vi "AuMT8852B Single Payload Use Dirty Tx.vi"(5 "Use Dirty transmitter? (F)":bool, 7 "Set/Get (Set)":enum16{"Set", "Get"}(ring), 8 "error in (no error)":errorcluster, 10 "Script (3)":i32=3, 11 "VISA session":refnum<visa-resource-name>) -> (0 "error out":errorcluster, 2 "error code":i32, 3 "VISA session out":refnum<visa-resource-name>, 4 "Use Dirty transmitter? out":bool)   [LabVIEW 2017]
doc: "Anritsu MT8852B Bluetooth Tester\n\nDetermines whether or not to use the Dirty Tx table for Bluetooth tests (Carrier, Sensitivity, etc.) whose scripts are set to Single Payload mode.\n\nINPUTS\nSet/Get - whether the value is being sent to or retrieved from the instrument.\nScript - the script to access.\nUse dirty transmitter? - value to be used in Single Payload mode.\n\nOUTPUTS\nUse dirty transmitter? out - value currently being used in Single Payload mode."
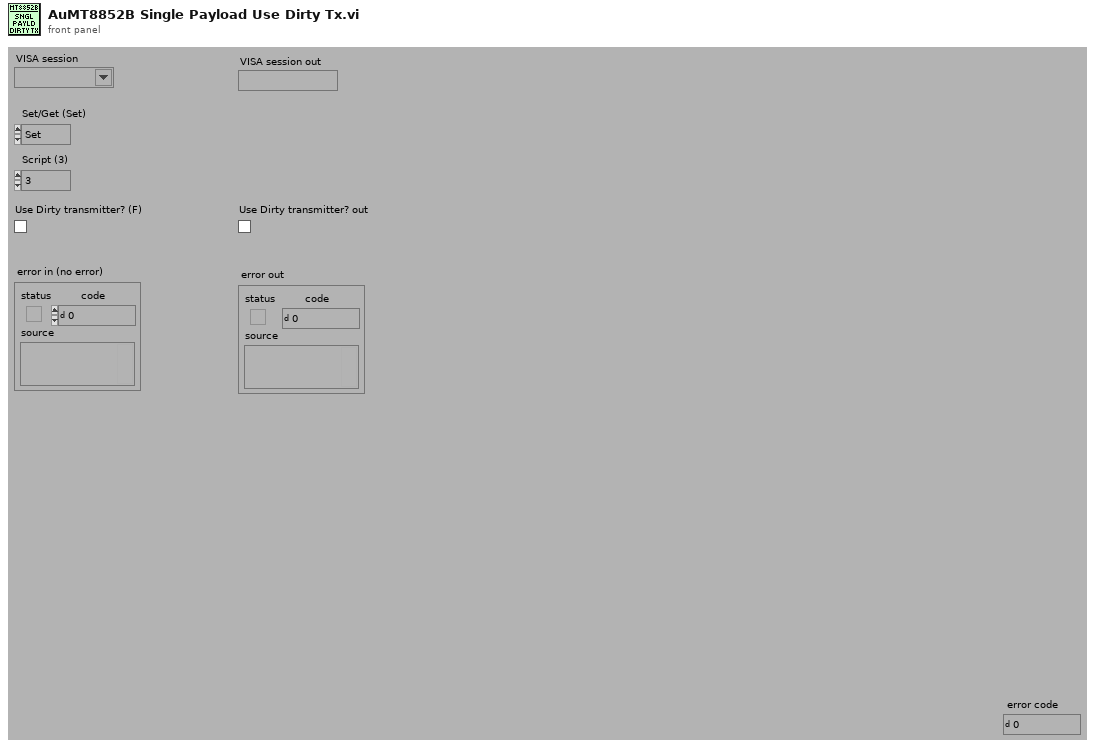
[diagram p1: front panel]
types:
  T1 = enum16{"Simulate", "Range check", "Cache", "Query instrument status"}
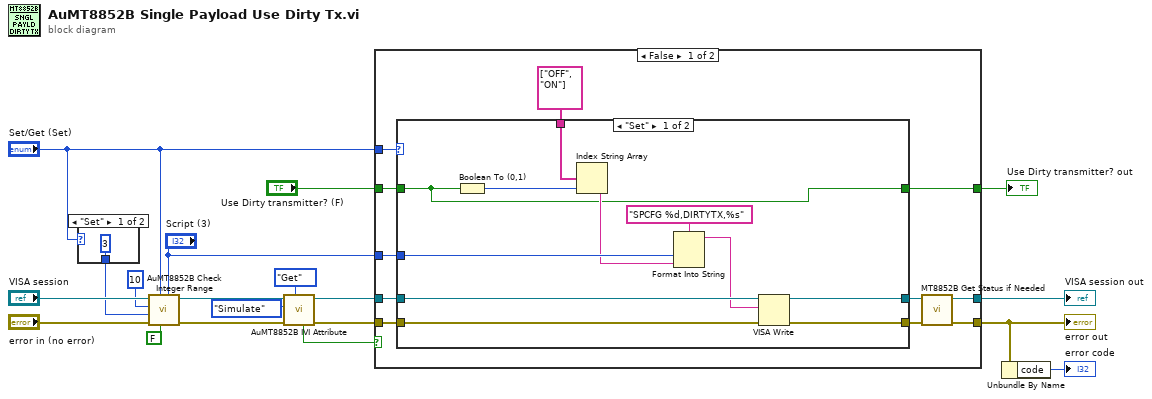
[diagram p0: block diagram]
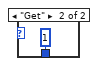
[diagram p2: hidden frame]
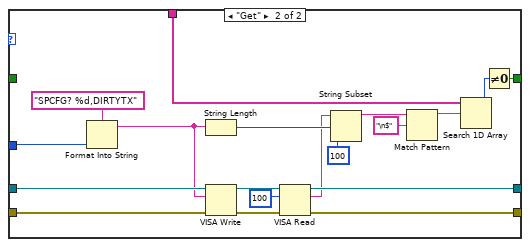
[diagram p3: hidden frame]
diagram:
  n1 = case shown="\"Set\"" "Set/Get (Set)" {
    tunnel: [3 1] -> w15
    frame "Set" {
    }
    frame "Get" {
    }
  }
  n2 = call <instrlib>:"AuMT8852B Check Integer Range.vi"("Value (0)"="Script (3)", "Check IVI flag first? (T)"=FALSE, "Set/Get (Set)"="Set/Get (Set)", "error in (no error)"="error in (no error)", "Lower limit (-1)"=w15, "Upper limit (1)"=10, "VISA session"="VISA session") -> ("error out"=w11:errorcluster, "VISA session out"=w14:refnum<visa-resource-name>)  [unwired: 3 in]
  n3 = call <instrlib>:"AuMT8852B IVI Attribute.vi"("Set/Get (Set)"=enum16{"Set", "Get"}."Get", "error in (no error)"=w11, "Flag (Simulate)"=T1."Simulate", "VISA session"=w14) -> ("error out"=w12:errorcluster, "VISA session out"=w13:refnum<visa-resource-name>, "Value out"=w8:bool)  [unwired: 5 in]
  n4 = case shown="False" w8 {
    tunnel: "Set/Get (Set)" -> [w32 _]
    tunnel: [w26 w64] -> w4
    tunnel: [w27 w65] -> w19
    tunnel: w13 -> [w31 w65]
    tunnel: w12 -> [w30 w64]
    tunnel: "Script (3)" -> [w25 _]
    tunnel: "Use Dirty transmitter? (F)" -> [w23 w63]
    tunnel: [w22 w63] -> w1
    frame False {
      n5 = case shown="\"Set\"" w32 {
        tunnel: [w40 w56] -> w28
        tunnel: [w41 w57] -> w29
        tunnel: w31 -> [w43 w62]
        tunnel: w30 -> [w42 w61]
        tunnel: w25 -> [w37 w54]
        tunnel: string[] ["OFF", "ON"] ("Array Constant") -> [w36 w46]
        tunnel: w23 -> [w33 _]
        tunnel: [w33 w44] -> w22
        frame "Set" {
          n6 = Boolean To (0,1)(Boolean=w33) -> (0, 1=w34:i16)
          n7 = Index String Array(1:w34, 2:w36) -> (0:w35:string)  [unwired: 1 in]
          n8 = Format Into String(format string="SPCFG %d,DIRTYTX,%s" ("Format String"), w37, w35) -> (resulting string=w38:string)  [unwired: 2 in, 1 out]
          n9 = VISA Write(VISA resource name=w43, write buffer=w38, error in (no error)=w42) -> (VISA resource name out=w41:refnum<visa-resource-name>, error out=w40:errorcluster)  [unwired: 1 out]
        }
        frame "Get" {
          n10 = Format Into String(format string="SPCFG? %d,DIRTYTX" ("Format String"), w54) -> (resulting string=w52:string)  [unwired: 2 in, 1 out]
          n11 = String Length(string=w52) -> (length=w51:i32)
          n12 = VISA Write(VISA resource name=w62, write buffer=w52, error in (no error)=w61) -> (VISA resource name out=w60:refnum<visa-resource-name>, error out=w58:errorcluster)  [unwired: 1 out]
          n13 = VISA Read(VISA resource name=w60, byte count=u32 100 ("byte count (0)"), error in (no error)=w58) -> (VISA resource name out=w57:refnum<visa-resource-name>, read buffer=w49:string, error out=w56:errorcluster)  [unwired: 1 out]
          n14 = String Subset(string=w49, offset (0)=w51, length (rest)=100 ("length (rest)")) -> (substring=w50:string)
          n15 = Match Pattern(string=w50, regular expression="\n$") -> (before substring=w47:string)  [unwired: 1 in, 3 out]
          n16 = Search 1D Array(1D array=w46, element=w47) -> (index of element=w45:i32)  [unwired: 1 in]
          n17 = Not Equal To 0?(x=w45) -> (x != 0?=w44:bool)
        }
      }
      n18 = call <instrlib>:"MT8852B Get Status if Needed.vi"("error in (no error)"=w28, "VISA session"=w29) -> ("error out"=w26:errorcluster, "VISA session out"=w27:refnum<visa-resource-name>)  [unwired: 8 in]
    }
    frame True {
    }
  }
  "error out" <- w4
  "VISA session out" <- w19
  "Use Dirty transmitter? out" <- w1
  n19 = Unbundle By Name(w4) -> ("code"=→"error code":i32)
